vi "Runtime Initialization Test.vi"() -> (0 "error out":errorcluster, 1 "Pass":bool, 2 "Tags Found":bool, 3 "Expected Execution Settings":bool)   [LabVIEW 2014, in "User Control Module Test.lvlib"]
doc: "Test that module can be initialized without any errors and that all channels are added to the appropriate data dictionary."
uses:
  User Control Module Test.lvlib
  module/execution/user control module.lvclass
  <vilib>/NI/Tag Bus/tag/tag descriptor.lvclass/tag descriptor.ctl
  <vilib>/NI/Tag Bus Module Framework/channel/TBM channel.lvclass/TBM channel.ctl
  <vilib>/NI/Tag Bus/tag/read tag name.vi
  <vilib>/NI/Tag Bus/tag/read data type.vi
  <vilib>/NI/Tag Bus Module Framework/channel/Read channel classification.vi
  module/configuration/user control module configuration.lvclass
  <vilib>/NI/Tag Bus/dictionary/data dictionary.lvclass
  <vilib>/NI/Tag Bus Module Framework/channel/TBM channel.lvclass
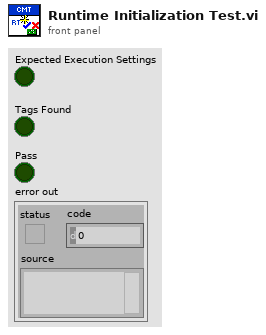
[diagram p1: front panel]
types:
  T1 = typedef "TBM channel.lvclass/data tables.ctl" = cluster{"input data":T2, "processing parameter":T2, "processing result":T2, "output data":T2}
  T2 = typedef "tag bus.lvlib/dictionary table pair.ctl" = cluster{"data dictionary":refnum<class "data dictionary.lvclass">, "data table":T3}
  T3 = typedef "tag bus.lvlib/data table.lvlib/data table.ctl" = cluster{"Double":dbl[], "Single":sgl[], "I64":i64[], "I32":i32[], "I16":i16[], "I8":i8[], "U64":u64[], "U32":u32[], "U16":u16[], "U8":u8[], "Boolean":bool[], "String":string[], "Array of Double":cluster{"DBL Array":dbl[]}[], "Array of Single":cluster{"SGL Array":sgl[]}[], "Array of I64":cluster{"I64 Array":i64[]}[], "Array of I32":cluster{"I32 Array":i32[]}[], "Array of I16":cluster{"I16 Array":i16[]}[], "Array of I8":cluster{"I8 Array":i8[]}[], "Array of U64":cluster{"U64 Array":u64[]}[], "Array of U32":cluster{"U32 Array":u32[]}[], "Array of U16":cluster{"U16 Array":u16[]}[], "Array of U8":cluster{"U8 Array":u8[]}[], "Array of Boolean":cluster{"Boolean Array":bool[]}[], "Array of String":cluster{"String Array":string[]}[]}
  T4 = typedef "TBM module execution interface.lvclass/execution settings.ctl" = cluster{"reads inputs":bool, "processes data":bool, "writes outputs":bool}
  T5 = typedef "tag bus.lvlib/tag descriptor.lvclass/Data Type.ctl" = enum16{"Double", "Single", "I64", "I32", "I16", "I8", "U64", "U32", "U16", "U8", "Boolean", "String", "Array of Double", "Array of Single", "Array of I64", "Array of I32", "Array of I16", "Array of I8", "Array of U64", "Array of U32", "Array of U16", "Array of U8", "Array of Boolean", "Array of String"}
  T6 = typedef "TBM channel.lvclass/channel classification.ctl" = enum16{"input data", "output data", "processing parameter", "processing result"}
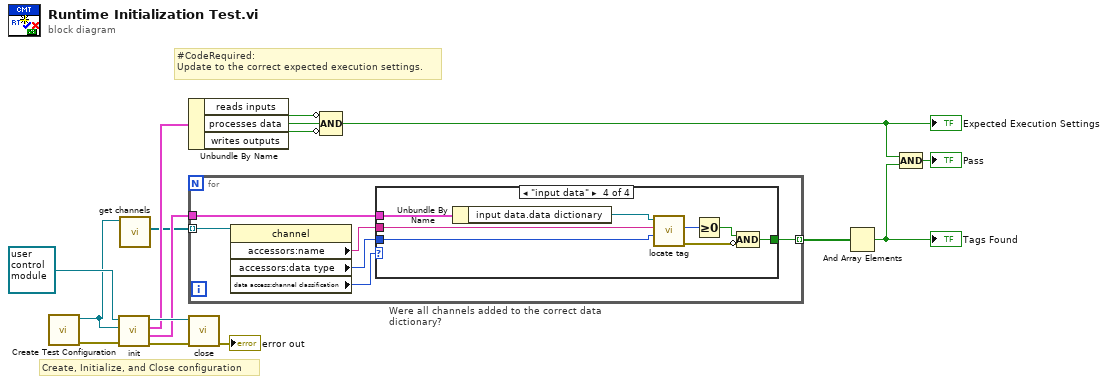
[diagram p0: block diagram]
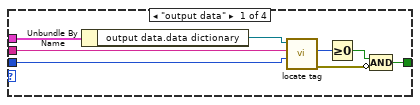
[diagram p2: hidden frame]
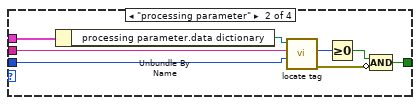
[diagram p3: hidden frame]
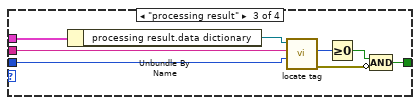
[diagram p4: hidden frame]
diagram:
  # "Create, Initialize, and Close configuration"
  # "#CodeRequired:\nUpdate to the correct expected execution settings."
  n1 = call "Create Test Configuration.vi"() -> ("error out"=w11:errorcluster, "Module"=w4:refnum<class "user control module configuration.lvclass">)  [unwired: 6 in, 4 out]
  n2 = call-dynamic "init.vi"("error in"=w11, "TBM module configuration in"=w4, "fixed channel runtime in"=refnum<class "user control module.lvclass"> refnum ("user module")) -> ("error out"=w9:errorcluster, "data allocations"=w8:T1, "execution settings"=w7:T4, "fixed channel runtime out"=w10:refnum<class "user control module.lvclass">)  [unwired: 5 in]
  n3 = call-dynamic "get channels.vi"("fixed channel configuration in"=w4) -> ("channels"=w6:refnum<class "TBM channel.lvclass">[])  [unwired: 9 in, 1 out]
  n4 = Unbundle By Name(w7) -> ("reads inputs"=w16:bool, "processes data"=w14:bool, "writes outputs"=w15:bool)
  n5 = for "Were all channels added to the correct data dictionary?" {
    tunnel: w8 -> [w22]
    tunnel: w6 -> [w21] mode=indexing
    tunnel: [w20] -> w13 mode=indexing
    n6 = property class="channel"(reference=w21) -> ("accessors:name"=w17:string, "accessors:data type"=w18:T5, "data access:channel classification"=w19:T6)  [unwired: 1 in, 2 out]
    n7 = case shown="\"input data\"" w19 {
      tunnel: w22 -> [w30 w38 w46 w54]
      tunnel: w18 -> [w28 w36 w44 w52]
      tunnel: w17 -> [w27 w35 w43 w51]
      tunnel: [w23 w31 w39 w47] -> w20
      frame "output data" {
        n8 = Unbundle By Name(w30) -> ("output data.data dictionary"=w29:refnum<class "data dictionary.lvclass">)
        n9 = call <vilib>:"locate tag.vi"("data type"=w28, "name"=w27, "data dictionary in"=w29) -> ("error out"=w24:errorcluster, "index"=w26:i32)  [unwired: 6 in, 1 out]
        n10 = Greater Or Equal To 0?(x=w26) -> (x >= 0?=w25:bool)
        n11 = Compound Arithmetic op=AND(w25, invert w24) -> (w23:bool)
      }
      frame "processing parameter" {
        n12 = Unbundle By Name(w38) -> ("processing parameter.data dictionary"=w37:refnum<class "data dictionary.lvclass">)
        n13 = call <vilib>:"locate tag.vi"("data type"=w36, "name"=w35, "data dictionary in"=w37) -> ("error out"=w32:errorcluster, "index"=w34:i32)  [unwired: 6 in, 1 out]
        n14 = Greater Or Equal To 0?(x=w34) -> (x >= 0?=w33:bool)
        n15 = Compound Arithmetic op=AND(w33, invert w32) -> (w31:bool)
      }
      frame "processing result" {
        n16 = Unbundle By Name(w46) -> ("processing result.data dictionary"=w45:refnum<class "data dictionary.lvclass">)
        n17 = call <vilib>:"locate tag.vi"("data type"=w44, "name"=w43, "data dictionary in"=w45) -> ("error out"=w40:errorcluster, "index"=w42:i32)  [unwired: 6 in, 1 out]
        n18 = Greater Or Equal To 0?(x=w42) -> (x >= 0?=w41:bool)
        n19 = Compound Arithmetic op=AND(w41, invert w40) -> (w39:bool)
      }
      frame "input data" {
        n20 = Unbundle By Name(w54) -> ("input data.data dictionary"=w53:refnum<class "data dictionary.lvclass">)
        n21 = call <vilib>:"locate tag.vi"("data type"=w52, "name"=w51, "data dictionary in"=w53) -> ("error out"=w48:errorcluster, "index"=w50:i32)  [unwired: 6 in, 1 out]
        n22 = Greater Or Equal To 0?(x=w50) -> (x >= 0?=w49:bool)
        n23 = Compound Arithmetic op=AND(w49, invert w48) -> (w47:bool)
      }
    }
  }
  n24 = call-dynamic "close.vi"("error in"=w9, "module in"=w10) -> ("error out"=→"error out":errorcluster)  [unwired: 9 in]
  n25 = Compound Arithmetic op=AND(invert w16, w14, invert w15) -> (w3:bool)
  "Expected Execution Settings" <- w3
  n26 = And Array Elements(Boolean array=w13) -> (logical AND=w2:bool)
  "Tags Found" <- w2
  n27 = Compound Arithmetic op=AND(w3, w2) -> (→"Pass":bool)
